vi "uActor_NestedStopped.vi"(8 "NestedActor - Last Error":errorcluster, 10 "NestedActor - Last State":refnum<class "uActor.lvclass">, 11 "uActor in":refnum<class "uActor.lvclass">) -> (0 "error out":errorcluster, 3 "uActor out":refnum<class "uActor.lvclass">)   [LabVIEW 2021, in "uFramework.lvlib" / "uActor.lvclass"]
doc: "Dynamic dispatch method that is called once a nested actor stops. This allows children to override the behavior of handling an incoming notification from a nested actor that it had closed.\n\nThe default behavior of the parent is to cascade up the error to the caller actor unless a child override is provided."
uses:
  uActor.lvclass
  uActor.lvclass/uActor.ctl
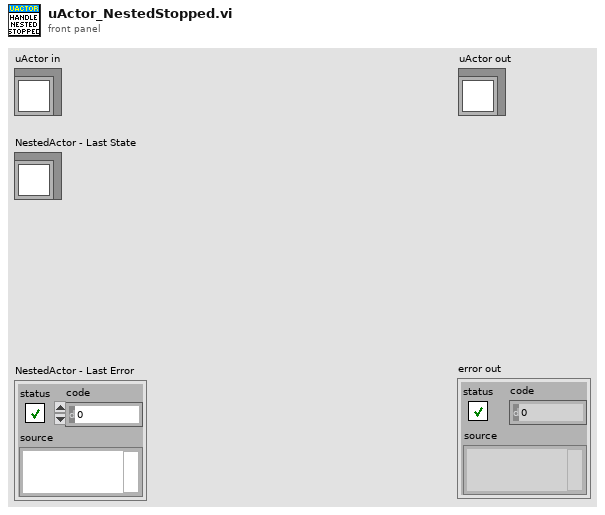
[diagram p1: front panel]
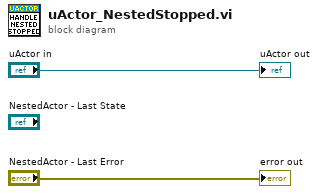
[diagram p0: block diagram]
diagram:
  "error out" <- "NestedActor - Last Error"
  "uActor out" <- "uActor in"
